vi "DefaultFromIni.vi"(8 "error in (no error)":errorcluster, 11 "MyPluginsBase in":refnum<class "NiDaqMx.lvclass">) -> (0 "error out":errorcluster, 3 "MyPluginsBase out":refnum<class "NiDaqMx.lvclass">)   [LabVIEW 2014, in "DigitizerPlugins.lvlib" / "NiDaqMx.lvclass"]
uses:
  NiDaqMx.lvclass
  SampleClock.ctl
  <userlib>/NIST/BaseClasses/BasePlugin_class/BasePlugin.lvclass/BasePlugin.ctl
  NiDaqMx.lvclass/NiDaqMx.ctl
  <userlib>/NIST/BaseClasses/BasePlugin_class/Accessors/Read PluginIniFilePath.vi
  Accessors/Write SampleClock.vi
  DigitizerBaseClass/DigitizerBase.lvclass
  <vilib>/Utility/config.llb/NI_LVConfig.lvlib
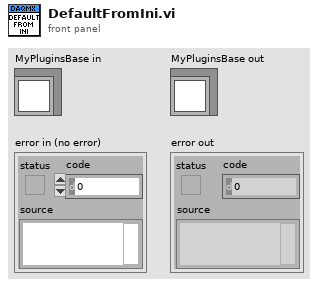
[diagram p1: front panel]
types:
  T1 = typedef "DigitizerPlugins.lvlib/NiDaqMx.lvclass/SampleClock.ctl" = cluster{"Type":enum16{"NULL", "Onboard", "External", "Software", "Interval"}, "Source":string, "TimebaseRate":dbl, "sample mode":i32}
  T2 = typedef "NI_LVConfig.lvlib/Config Data RefNum.ctl" = refnum<k1>
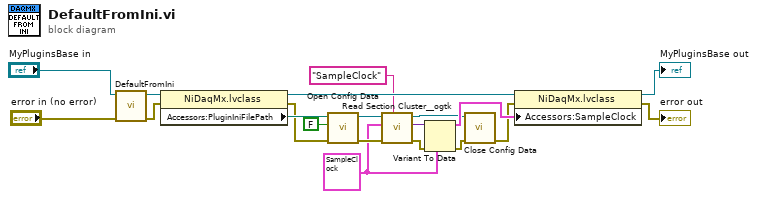
[diagram p0: block diagram]
diagram:
  w7 = T1 {"Type"=enum."NULL", "Source"="", "TimebaseRate"=18000000.0, "sample mode"=10123} ("SampleClock")
  n1 = call-parent "DefaultFromIni.vi"("error in (no error)"="error in (no error)", "MyPluginsBase in"="MyPluginsBase in") -> ("error out"=w16:errorcluster, "MyPluginsBase out"=w20:refnum<class "NiDaqMx.lvclass">)  [unwired: 8 in]
  n2 = property class="NiDaqMx.lvclass"(reference=w20, error in=w16) -> (reference out=w17:refnum<class "NiDaqMx.lvclass">, error out=w13:errorcluster, "Accessors:PluginIniFilePath"=w15:path)
  n3 = call <vilib>:"Open Config Data.vi"("error in (no error)"=w13, "create file if necessary (T)"=FALSE, "configuration file path"=w15) -> ("error out"=w11:errorcluster, "refnum"=w10:T2)  [unwired: 6 in, 1 out]
  n4 = call <userlib>:"Read Section Cluster__ogtk.vi"("section (optional)"="SampleClock", "error in (no error)"=w11, "Section Formatted Cluster Type"=w7, "refnum"=w10) -> ("error out"=w6:errorcluster, "Section Formatted Cluster"=w8:variant, "dup refnum"=w3:T2)  [unwired: 3 in, 2 out]
  n5 = Variant To Data(error in=w6, type=w7, Variant=w8) -> (data=w5:T1, error out=w4:errorcluster)
  n6 = call <vilib>:"Close Config Data.vi"("error in (no error)"=w4, "refnum"=w3) -> ("error out"=w2:errorcluster)  [unwired: 8 in, 1 out]
  n7 = property class="NiDaqMx.lvclass"(reference=w17, error in=w2, "Accessors:SampleClock"=w5) -> (reference out=→"MyPluginsBase out":refnum<class "NiDaqMx.lvclass">, error out=→"error out":errorcluster)
